vi "checkFinishNormalGamePlayVSS.vi"(8 "error in (no error)":errorcluster, 9 "last command_interpreted":T1, 10 "Game in":refnum<class "Game.lvclass">, 11 "NormalGamePlayVSS in":refnum<class "NormalGamePlayVSS.lvclass">) -> (0 "error out":errorcluster, 2 "Boolean":bool, 3 "NormalGamePlayVSS out":refnum<class "NormalGamePlayVSS.lvclass">)   [LabVIEW 2018, in "NormalGamePlayVSS.lvclass"]
uses:
  NormalGamePlayVSS.lvclass
  Game_class/Game.lvclass
  Referee_class/command_interpreted.ctl
  Game_class/Game.lvclass/Game.ctl
  Referee_class/Referee.lvclass/Referee.ctl
  Events_class/Events.lvclass/Events.ctl
  Game_class/Read Referee.vi
  Game_class/Read EventsRef.vi
  Events_class/Read ball_out_of_vision.vi
  Events_class/Read ball_out.vi
  Referee_class/Read command_interpreted.vi
  Referee_class/Referee.lvclass
  Events_class/Events.lvclass
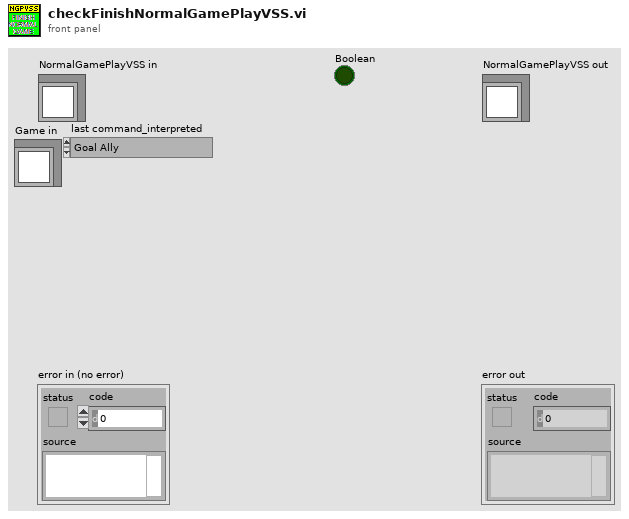
[diagram p1: front panel]
types:
  T1 = typedef "command_interpreted.ctl" = enum16{"Goal Ally", "Goal Enemy", "Ball Placement Enemy", "Ball Placement Ally", "Normal Half Time", "Extra Time  Break", "Extra Half Time", "None", "Post Game", "PKA Normal Start", "Prepare Kickoff Ally", "PKE Normal Start", "Prepare Kickoff Enemy", "Force Start", "Halt", "Timeout", "Prepare Penalty Ally", "Prepare Penalty Enemy", "PPA NormalStart", "PPE Normal Start", "Indirect Free Ally", "Direct Free Enemy", "Direct Free Ally", "Indirect Free Enemy", "Stop"}
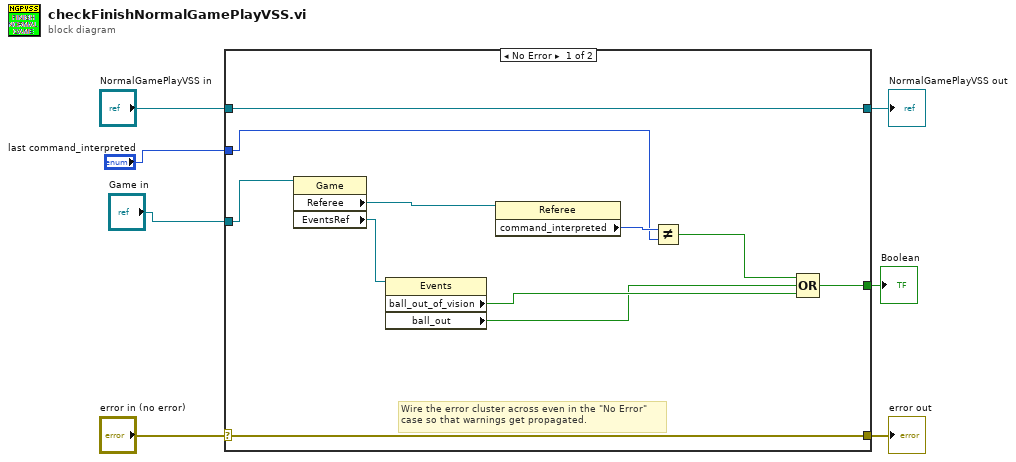
[diagram p0: block diagram]
diagram:
  n1 = case shown="No Error" "error in (no error)" {
    selector: "error in (no error)" -> [w17 w20]
    tunnel: [w17 w20] -> w6
    tunnel: [w18 w19] -> w4
    tunnel: "NormalGamePlayVSS in" -> [w18 w19]
    tunnel: "Game in" -> [w10 _]
    tunnel: "last command_interpreted" -> [w9 _]
    tunnel: [w8 _] -> w1
    frame No Error {
      # "Wire the error cluster across even in the \"No Error\"\ncase so that warnings get propagated."
      n2 = property class="Game"(reference=w10) -> ("Referee"=w16:refnum<class "Referee.lvclass">, "EventsRef"=w14:refnum<class "Events.lvclass">)  [unwired: 1 in, 2 out]
      n3 = property class="Events"(reference=w14) -> ("ball_out_of_vision"=w12:bool, "ball_out"=w11:bool)  [unwired: 1 in, 2 out]
      n4 = property class="Referee"(reference=w16) -> ("command_interpreted"=w15:T1)  [unwired: 1 in, 2 out]
      n5 = Not Equal?(x=w15, y=w9) -> (x != y?=w13:bool)
      n6 = Compound Arithmetic op=OR(w13, w11, w12) -> (w8:bool)
    }
    frame Error {
    }
  }
  "error out" <- w6
  "NormalGamePlayVSS out" <- w4
  "Boolean" <- w1
